vi "roboRIO Read Default State.vi"(7 "Size":i32, 8 "error in":errorcluster, 9 "Path":path, 11 "Connector":string) -> (0 "error out":errorcluster, 2 "Default Connector Info":string[](array[string]), 3 "Default Pins IDs":string[](array[string]))   [LabVIEW 2021]
doc: "This VI reads Pin name from \"Config.ini\" based on Connector Type,\nPin Peripheral and Pin Number."
uses:
  <vilib>/Utility/config.llb/Read Key (String).vi
  <vilib>/Utility/config.llb/NI_LVConfig.lvlib
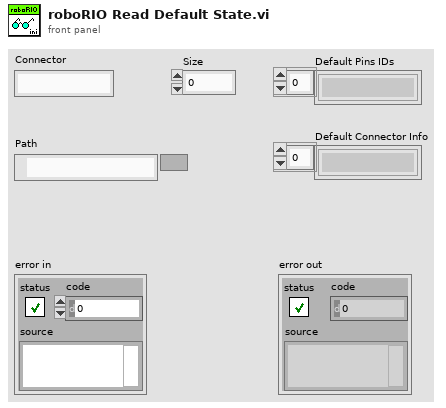
[diagram p1: front panel]
types:
  T1 = typedef "NI_LVConfig.lvlib/Config Data RefNum.ctl" = refnum<k1>
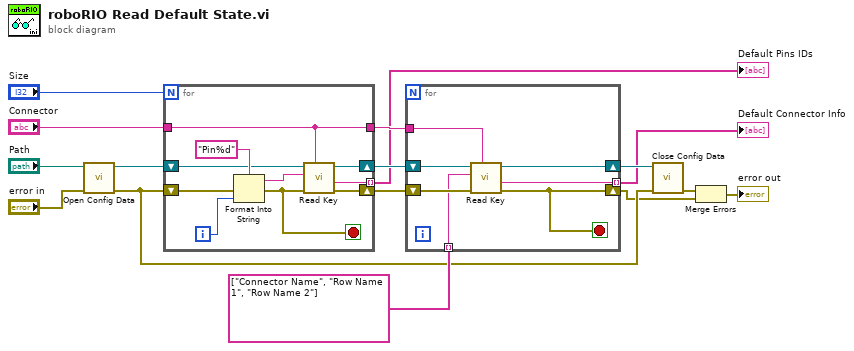
[diagram p0: block diagram]
diagram:
  n1 = call <vilib>:"Open Config Data.vi"("error in (no error)"="error in", "configuration file path"="Path") -> ("error out"=w5:errorcluster, "refnum"=w16:T1)  [unwired: 7 in, 1 out]
  n2 = for {
    N: "Size" -> [_]
    shift-right: [w22] -> w7
    shift-left: w5 -> [w21]
    shift-right: [w23] -> w9
    shift-left: w16 -> [w24]
    tunnel: [w20] -> w2 mode=indexing
    tunnel: "Connector" -> [w18]
    tunnel: [w18] -> w8
    i -> [w17]
    stop <- w19 stop-if-true
    n3 = Format Into String(format string="Pin%d", error in=w21, w17) -> (resulting string=w26:string, error out=w19:errorcluster)  [unwired: 1 in]
    n4 = call-poly <vilib>:"Read Key.vi"("section"=w18, "error in (no error)"=w19, "key"=w26, "refnum"=w24) -> ("error out"=w22:errorcluster, "value"=w20:string, "refnum out"=w23:T1)  [unwired: 4 in, 1 out]
  }
  "Default Pins IDs" <- w2
  n5 = for {
    shift-right: [w28] -> w4
    shift-left: w9 -> [w31]
    tunnel: w8 -> [w33]
    shift-right: [w27] -> w3
    shift-left: w7 -> [w32]
    tunnel: string[] ["Connector Name", "Row Name 1", "Row Name 2"] -> [w30] mode=indexing
    tunnel: [w29] -> w1 mode=indexing
    stop <- w27 stop-if-true
    n6 = call-poly <vilib>:"Read Key.vi"("section"=w33, "error in (no error)"=w32, "key"=w30, "refnum"=w31) -> ("error out"=w27:errorcluster, "value"=w29:string, "refnum out"=w28:T1)  [unwired: 4 in, 1 out]
  }
  "Default Connector Info" <- w1
  n7 = call <vilib>:"Close Config Data.vi"("error in (no error)"=w5, "refnum"=w4) -> ("error out"=w11:errorcluster)  [unwired: 8 in, 1 out]
  n8 = Merge Errors(w11, w3) -> (→"error out":errorcluster)
